vi "NI VeriStand - Get Item Children.vi"(8 "error in (no error)":errorcluster, 11 "Item Ref in":T1 format="%.0x") -> (0 "error out":errorcluster, 2 "Child Refs":T1[](array[typedef]) format="%.0x", 3 "Item Ref out":T1 format="%.0x", 4 "Found":bool)   [LabVIEW 2019, in "Custom Device API.lvlib"]
doc: "Returns a list of references to all child items of the item specified by <B>Item Ref in</B>. This list can include subsections and channels."
uses:
  Custom Device API.lvlib
  Custom Device Item Ref.ctl
  Custom Device Offline Path.vi
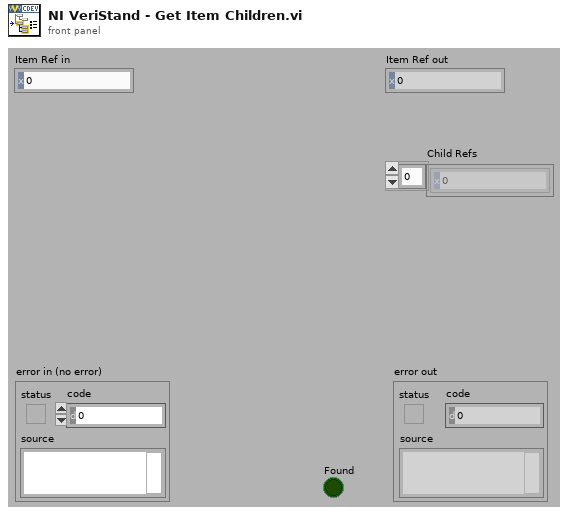
[diagram p1: front panel]
types:
  T1 = typedef "Custom Device API.lvlib/Custom Device Item Ref.ctl" = u64
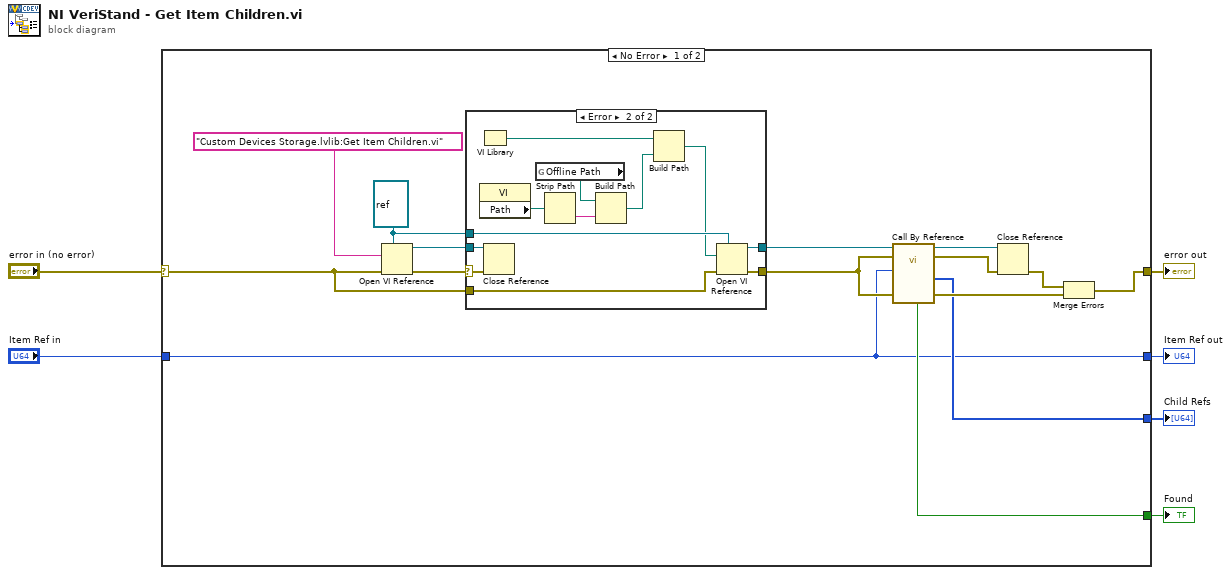
[diagram p0: block diagram]
diagram:
  n1 = case shown="No Error" "error in (no error)" {
    selector: "error in (no error)" -> [w8 w36]
    tunnel: [w16 w36] -> w6
    tunnel: "Item Ref in" -> [w7 w37]
    tunnel: [w7 w37] -> w4
    tunnel: [w15 _] -> w3
    tunnel: [w14 _] -> w2
    frame No Error {
      w11 = refnum<vi> refnum ("type specifier VI Refnum (for type only)")
      n2 = Open VI Reference(type specifier VI Refnum (for type only)=w11, vi path="Custom Devices Storage.lvlib:Get Item Children.vi", error in (no error)=w8) -> (vi reference=w12:refnum<vi>, error out=w13:errorcluster)  [unwired: 3 out]
      n3 = case shown="Error" w13 {
        selector: w13 -> [w22 w32]
        tunnel: w11 -> [_ w34]
        tunnel: w12 -> [w23 w33]
        tunnel: [w23 w31] -> w9
        tunnel: [w22 w30] -> w10
        tunnel: w8 -> [_ w35]
        frame No Error {
        }
        frame Error {
          n4 = VI Library() -> (path=w29:path)
          n5 = property class="VI"() -> ("Path"=w25:path)  [unwired: 2 in, 2 out]
          n6 = Close Reference(reference=w33, error in (no error)=w32) -> ()  [unwired: 1 out]
          n7 = global read "Custom Device Offline Path.vi" "Offline Path"() -> (w26:path)
          n8 = Strip Path(path=w25) -> (name=w24:string)  [unwired: 1 out]
          n9 = Build Path(base path=w26, name or relative path=w24) -> (appended path=w28:path)
          n10 = Build Path(base path=w29, name or relative path=w28) -> (appended path=w27:path)
          n11 = Open VI Reference(type specifier VI Refnum (for type only)=w34, vi path=w27, error in (no error)=w35) -> (vi reference=w31:refnum<vi>, error out=w30:errorcluster)  [unwired: 3 out]
        }
      }
      n12 = call-by-ref "?"(reference=w9, error in=w10, 8:"error in (no error)"=w10, "Item Ref in"=w7) -> (reference out=w18:refnum<vi>, error out=w19:errorcluster, 0:"error out"=w20:errorcluster, "Child Refs"=w15:T1[], "Found"=w14:bool)  [unwired: 6 in, 1 out]
      n13 = Close Reference(reference=w18, error in (no error)=w19) -> (error out=w17:errorcluster)
      n14 = Merge Errors(w17, w20) -> (w16:errorcluster)
    }
    frame Error {
    }
  }
  "Item Ref out" <- w4
  "error out" <- w6
  "Found" <- w2
  "Child Refs" <- w3
